vi "Load 5668 FPGA Personality and Parameters.vi"(0 "Start Carrier Frequency in":dbl=1.0 format="%#_6p", 11 "error in":errorcluster) -> (4 "IQ rate (S/s)":dbl, 6 "option string":string, 8 "Signal Path:IF Filter Bandwidth":dbl, 10 "Spacing Center Frequencies":dbl, 15 "error out":errorcluster)   [LabVIEW 2017]
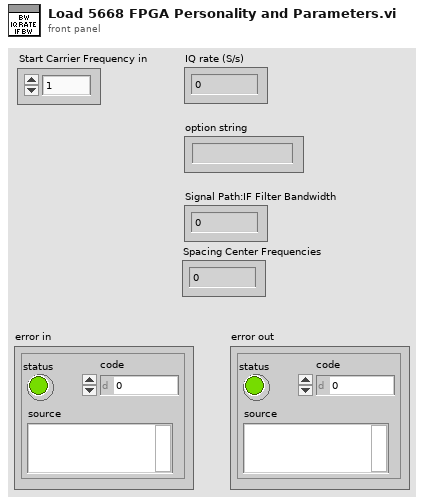
[diagram p1: front panel]
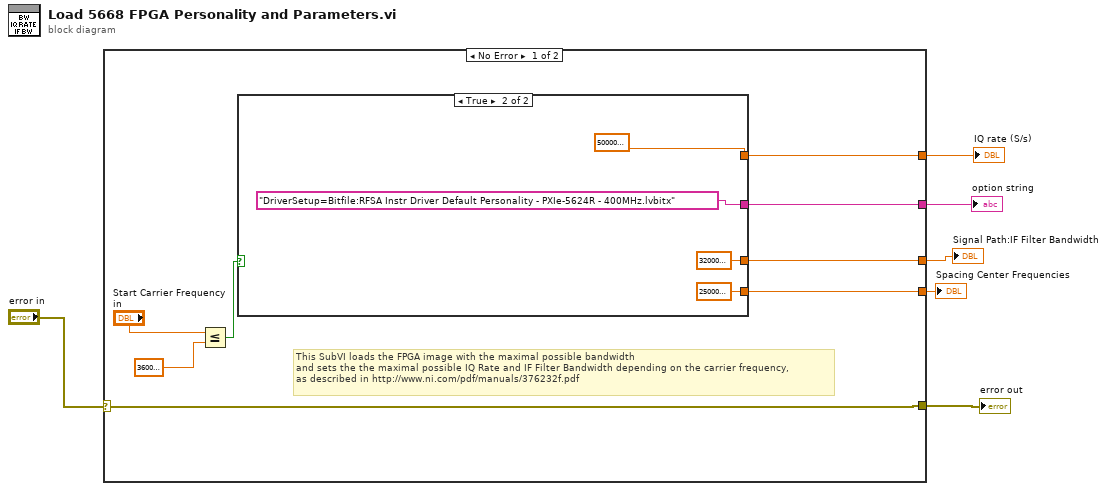
[diagram p0: block diagram]
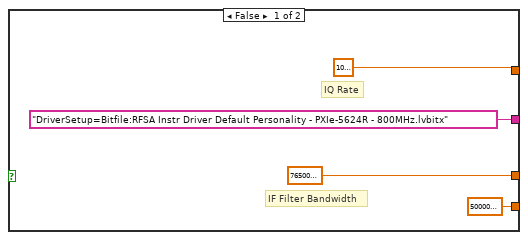
[diagram p2: hidden frame]
diagram:
  n1 = case shown="No Error" "error in" {
    selector: "error in" -> [w8 w23]
    tunnel: [w14 _] -> w6
    tunnel: [w11 _] -> w5
    tunnel: [w9 _] -> w4
    tunnel: [w8 w23] -> w2
    tunnel: [w7 _] -> w1
    frame No Error {
      # "This SubVI loads the FPGA image with the maximal possible bandwidth \nand sets the the maximal possible IQ Rate and IF Filter Bandwidth depending on the carrier frequency, \nas described in http://www.ni.com/pdf/manuals/376232f.pdf"
      n2 = Less Or Equal?(x="Start Carrier Frequency in", y=3600000000.0) -> (x <= y?=w13:bool)
      n3 = case shown="True" w13 {
        tunnel: ["DriverSetup=Bitfile:RFSA Instr Driver Default Personality - PXIe-5624R - 800MHz.lvbitx" ("option string") "DriverSetup=Bitfile:RFSA Instr Driver Default Personality - PXIe-5624R - 400MHz.lvbitx" ("option string")] -> w9
        tunnel: [765000000.0 ("Signal Path:IF Filter Bandwidth") 320000000.0 ("Signal Path:IF Filter Bandwidth")] -> w11
        tunnel: [1000000000.0 ("IQ rate (S/s)") 500000000.0 ("IQ rate (S/s)")] -> w14
        tunnel: [500000000.0 ("Signal Path:IF Filter Bandwidth") 250000000.0 ("Signal Path:IF Filter Bandwidth")] -> w7
        frame False {
          # "IF Filter Bandwidth"
          # "IQ Rate"
        }
        frame True {
        }
      }
    }
    frame Error {
    }
  }
  "IQ rate (S/s)" <- w6
  "Signal Path:IF Filter Bandwidth" <- w5
  "option string" <- w4
  "error out" <- w2
  "Spacing Center Frequencies" <- w1
